vi "FTW-TransferClient-UploadBegin.vi"(0 "Transfer Client":refnum<k24>, 5 "Remote URI":string, 7 "Local Filepath":path, 11 "error in":errorcluster) -> (4 "Transfer Client out":refnum<k24>, 6 "Upload Events":refnum<event-registration>, 15 "error out":errorcluster)   [LabVIEW 2015]
uses:
  FTW-TransferClient-TransferProgress.ctl
  FTW-TransferClient-TransferStatus.ctl
panel:
  # "Inputs"
  # "Outputs"
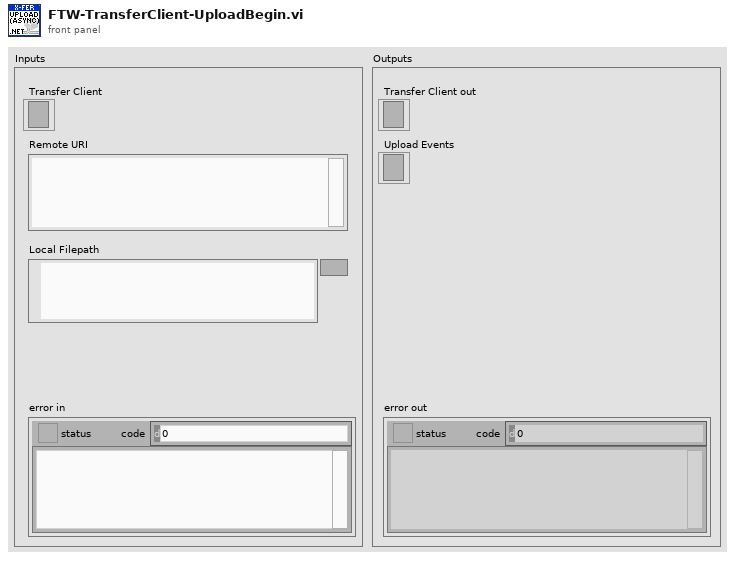
[diagram p1: front panel]
types:
  T1 = cluster{"Transfer Complete":refnum<user-event>, "Current Time":dbl, "AbsoluteURI":string, "Local Filepath":path}
  T2 = cluster{"Transfer Progress":refnum<user-event>, "Current Time":dbl, "AbsoluteURI":string, "Local Filepath":path}
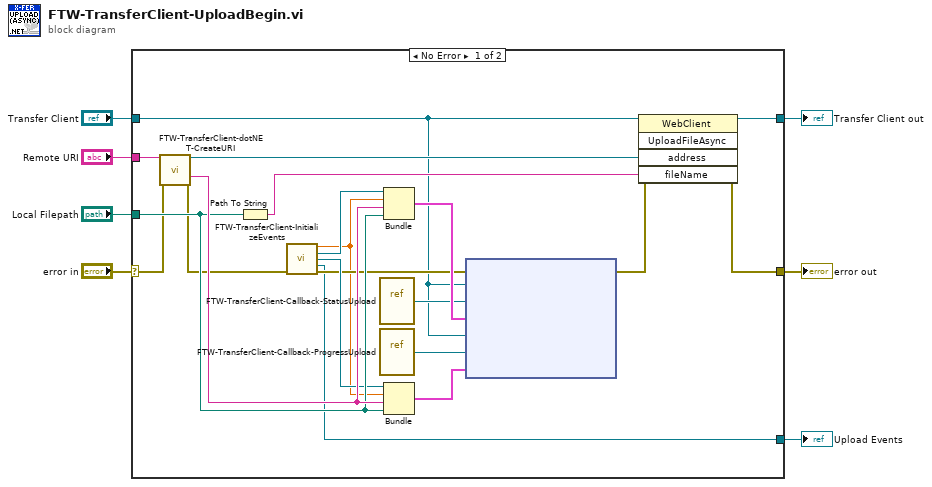
[diagram p0: block diagram]
diagram:
  n1 = case shown="No Error" "error in" {
    selector: "error in" -> [w23 w28]
    tunnel: "Transfer Client" -> [w9 w29]
    tunnel: [w22 w28] -> w6
    tunnel: [w8 w29] -> w7
    tunnel: "Local Filepath" -> [w24 _]
    tunnel: [w12 _] -> w5
    tunnel: "Remote URI" -> [w10 _]
    frame No Error {
      n2 = call "FTW-TransferClient-dotNET-CreateURI.vi"("URI"=w10, "error in"=w23) -> ("URI ref"=w26:refnum<k24>, "AbsoluteURI"=w25:string, "error out"=w14:errorcluster)  [unwired: 8 in, 3 out]
      n3 = Path To String(path=w24) -> (string=w27:string)
      n4 = call "FTW-TransferClient-InitializeEvents.vi"("error in"=w14) -> ("Current Time"=w11:dbl, "Transfer Complete"=w15:refnum<user-event>, "Transfer Progress"=w16:refnum<user-event>, "Transfer Events"=w12:refnum<event-registration>, "error out"=w13:errorcluster)  [unwired: 10 in]
      n5 = vi-ref "FTW-TransferClient-Callback-StatusUpload.vi"() -> ("vi reference"=w18:refnum<vi>)
      n6 = vi-ref "FTW-TransferClient-Callback-ProgressUpload.vi"() -> ("vi reference"=w17:refnum<vi>)
      n7 = Bundle("Transfer Complete"=w15, "Current Time"=w11, "AbsoluteURI"=w25, "Local Filepath"=w24) -> (w19:T1)  [unwired: 1 in]
      n8 = Bundle("Transfer Progress"=w16, "Current Time"=w11, "AbsoluteURI"=w25, "Local Filepath"=w24) -> (w21:T2)  [unwired: 1 in]
      n9 = node(w13, w9, w18, w19, w9, w17, w21) -> (w20:errorcluster)  [unwired: 1 in, 1 out]
      n10 = invoke class="WebClient" method="UploadFileAsync"(reference=w9, error in=w20, "address"=w26, "fileName"=w27) -> (reference out=w8:refnum<k24>, error out=w22:errorcluster)  [unwired: 1 in, 3 out]
    }
    frame Error {
    }
  }
  "error out" <- w6
  "Transfer Client out" <- w7
  "Upload Events" <- w5
